vi "Resume.vi"(8 "error in (no error)":errorcluster, 11 "Sequence in":refnum<class "Sequence.lvclass">) -> (0 "error out":errorcluster, 1 "TestSeqResumed":bool, 3 "Sequence out":refnum<class "Sequence.lvclass">)   [LabVIEW 2018, in "Sequence.lvclass"]
uses:
  Sequence.lvclass
  Sequence.lvclass/Sequence.ctl
  Support/MessageAPI/UIMessage.ctl
  SendMessage/SendMessage.lvclass
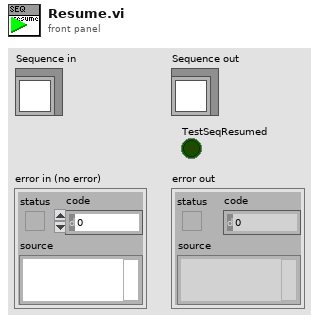
[diagram p1: front panel]
types:
  T1 = typedef "UIMessage.ctl" = cluster{"EventCode":i32, "Numeric":dbl, "String":string, "Variant":variant}
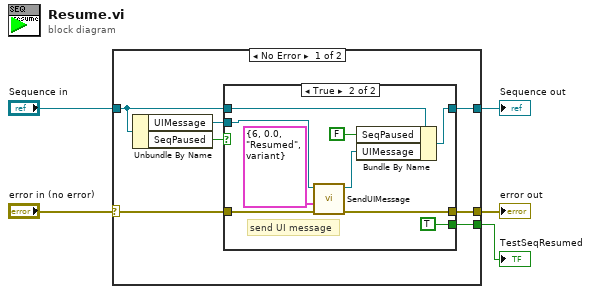
[diagram p0: block diagram]
diagram:
  n1 = case shown="No Error" "error in (no error)" {
    selector: "error in (no error)" -> [w7 w25]
    tunnel: [w6 w25] -> w2
    tunnel: [w9 w24] -> w3
    tunnel: "Sequence in" -> [w10 w24]
    tunnel: [w11 _] -> w1
    frame No Error {
      n2 = Unbundle By Name(w10) -> ("UIMessage"=w8:refnum<class "SendMessage.lvclass">, "SeqPaused"=w12:bool)
      n3 = case shown="True" w12 {
        tunnel: [_ TRUE] -> w11
        tunnel: [w14 w22] -> w9
        tunnel: w10 -> [w14 w23]
        tunnel: w8 -> [_ w18]
        tunnel: w7 -> [w13 w17]
        tunnel: [w13 w16] -> w6
        frame False {
        }
        frame True {
          # "send UI message"
          n4 = call-dynamic "SendUIMessage.vi"("error in (no error)"=w17, "UIMsg"=T1 {"EventCode"=6, "Numeric"=0.0, "String"="Resumed", "Variant"=variant}, "SendMessage in"=w18) -> ("error out"=w16:errorcluster, "SendMessage out"=w15:refnum<class "SendMessage.lvclass">)  [unwired: 7 in]
          n5 = Bundle By Name(cluster=w23, "SeqPaused"=FALSE, "UIMessage"=w15) -> (w22:refnum<class "Sequence.lvclass">)
        }
      }
    }
    frame Error {
    }
  }
  "error out" <- w2
  "Sequence out" <- w3
  "TestSeqResumed" <- w1
